vi "Check if existing column.vi"(5 "Init":bool, 7 "New Heading":string[](array[string]), 10 "New Data":string[][](array[string]), 11 "Main Heading in":string[](array[string])) -> (2 "New Data out":string[][](array[string]), 3 "Main Heading":string[](array[string]))   [LabVIEW 2020]
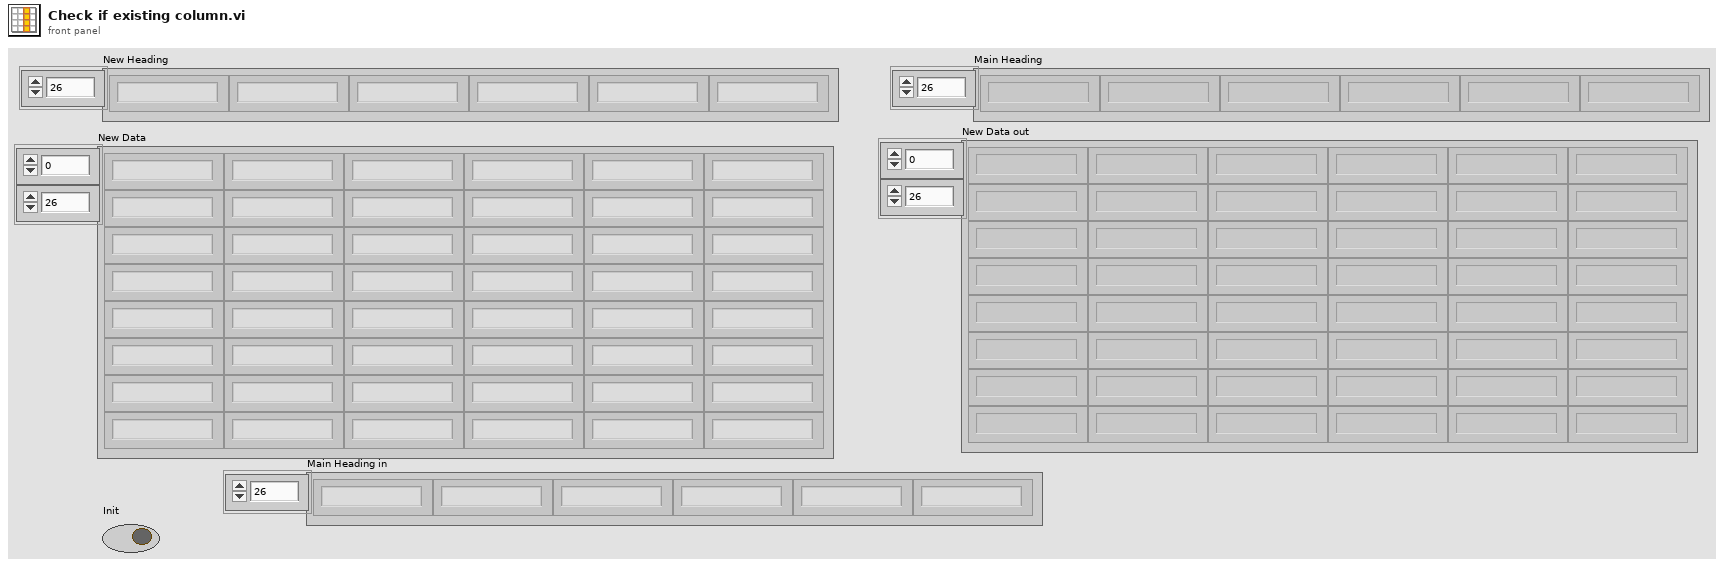
[diagram p1: front panel]
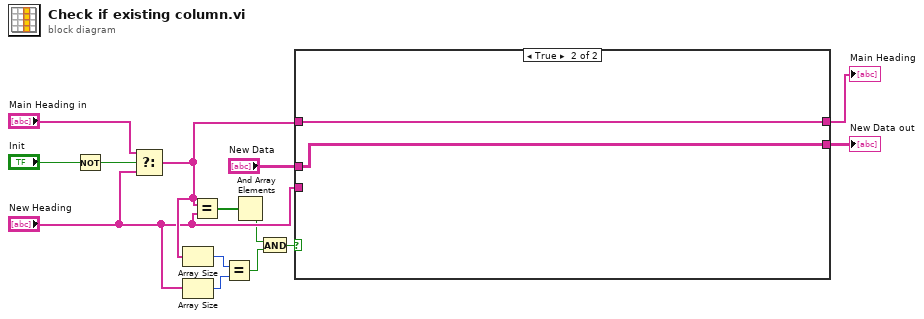
[diagram p0: block diagram]
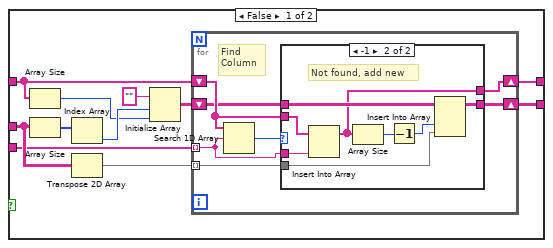
[diagram p2: hidden frame]
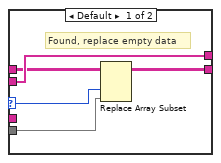
[diagram p3: hidden frame]
diagram:
  n1 = Not(x="Init") -> (.not. x?=w9:bool)
  n2 = Select(t="Main Heading in", s=w9, f="New Heading") -> (s? t:f=w7:string[])
  n3 = Array Size(array=w7) -> (size(s)=w4:i32)
  n4 = Array Size(array="New Heading") -> (size(s)=w5:i32)
  n5 = Equal?(x=w7, y="New Heading") -> (x = y?=w11:bool[])
  n6 = Equal?(x=w4, y=w5) -> (x = y?=w3:bool)
  n7 = And Array Elements(Boolean array=w11) -> (logical AND=w2:bool)
  n8 = And(x=w2, y=w3) -> (x .and. y?=w1:bool)
  n9 = case shown="True" w1 {
    tunnel: [w25 w47] -> w14
    tunnel: [w24 w46] -> w13
    tunnel: "New Data" -> [w19 w46]
    tunnel: w7 -> [w16 w47]
    tunnel: "New Heading" -> [w15 _]
    frame False {
      n10 = Array Size(array=w16) -> (size(s)=w17:i32)
      n11 = Array Size(array=w19) -> (size(s)=w22:i32[])
      n12 = Index Array(array=w22) -> (element=w21:i32)  [unwired: 1 in]
      n13 = Transpose 2D Array(2D array=w19) -> (transposed array=w18:string[][])
      n14 = Initialize Array("", w21, w17) -> (w20:string[][])
      n15 = for {
        tunnel: w15 -> [w31] mode=indexing
        tunnel: w18 -> [w28] mode=indexing
        shift-right: [w30] -> w25
        shift-left: w16 -> [w32]
        shift-right: [w26] -> w24
        shift-left: w20 -> [w29]
        # "Find\nColumn"
        n16 = Search 1D Array(1D array=w32, element=w31) -> (index of element=w27:i32)  [unwired: 1 in]
        n17 = case shown="-1" w27 {
          selector: w27 -> [w33 _]
          tunnel: w32 -> [w37 w45]
          tunnel: w31 -> [_ w44]
          tunnel: [w37 w41] -> w30
          tunnel: w29 -> [w36 w43]
          tunnel: w28 -> [w35 w39]
          tunnel: [w34 w42] -> w26
          frame Default {
            # "Found, replace empty data"
            n18 = Replace Array Subset(array=w36, new element=w35, index (col)=w33) -> (w34:string[][])  [unwired: 1 in]
          }
          frame -1 {
            # "Not found, add new"
            n19 = Insert Into Array(array=w45, new element=w44) -> (w41:string[])  [unwired: 1 in]
            n20 = Array Size(array=w41) -> (size(s)=w40:i32)
            n21 = Decrement(x=w40) -> (x-1=w38:i32)
            n22 = Insert Into Array(array=w43, index (col)=w38, new element=w39) -> (w42:string[][])  [unwired: 1 in]
          }
        }
      }
    }
    frame True {
    }
  }
  "Main Heading" <- w14
  "New Data out" <- w13
